vi "Add_Post_Install_Step.vi"(8 "error in (no error)":errorcluster, 11 "IB_Source in":refnum<class "IB_Source.lvclass">) -> (0 "error out":errorcluster, 1 "add?":bool, 2 "Pre_Uninstall_Step":refnum<class "IB_Post_Install_Step.lvclass">, 3 "Post_Install_Step":refnum<class "IB_Post_Install_Step.lvclass">)   [LabVIEW 2020, in "IB_Source.lvclass"]
uses:
  <vilib>/AppBuilder/IB_Classes/Source/IB_Source.lvclass
  <vilib>/AppBuilder/IB_Classes/Source/IB_Source.lvclass/IB_Source.ctl
  <vilib>/AppBuilder/IB_Classes/Post_Install_Step/IB_Post_Install_Step.lvclass
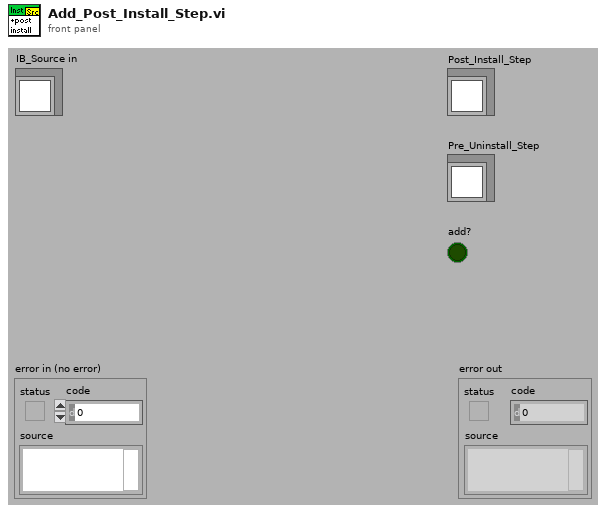
[diagram p1: front panel]
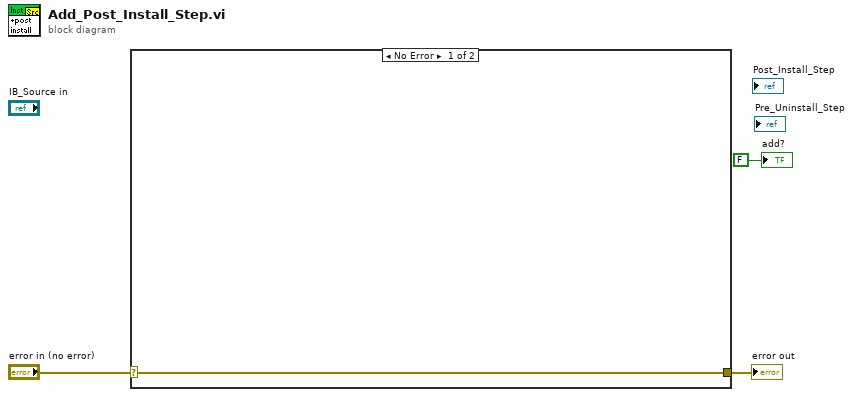
[diagram p0: block diagram]
diagram:
  n1 = case shown="No Error" "error in (no error)" {
    selector: "error in (no error)" -> [w4 w5]
    tunnel: [w4 w5] -> w2
    frame No Error {
    }
    frame Error {
    }
  }
  "error out" <- w2
  "add?" <- FALSE ("add?")
